vi "Example Test 3.vi"() -> ()   [LabVIEW 2014]
uses:
  <vilib>/measure/NI_MABase.lvlib
panel:
  out "error out 2":errorcluster
  out "myString":string
  out "signal out 2":waveform(dbl)
  in  "b 2":dbl=4.0
  in  "a 2":dbl=3.0
  out "signal out":waveform(dbl)
  out "error out":errorcluster
  in  "error in (no error)":errorcluster
  in  "b":dbl=2.0
  in  "a":dbl=1.0
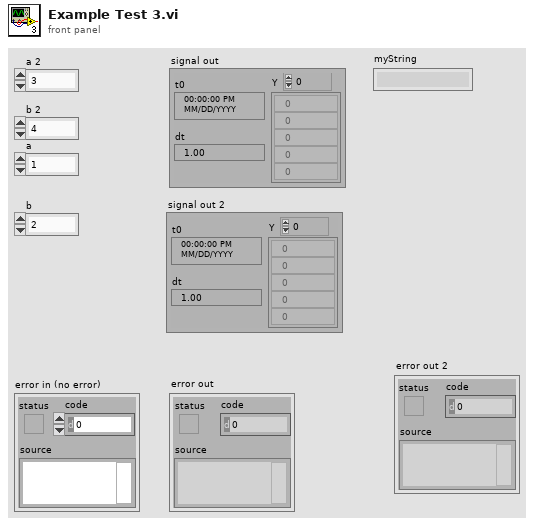
[diagram p1: front panel]
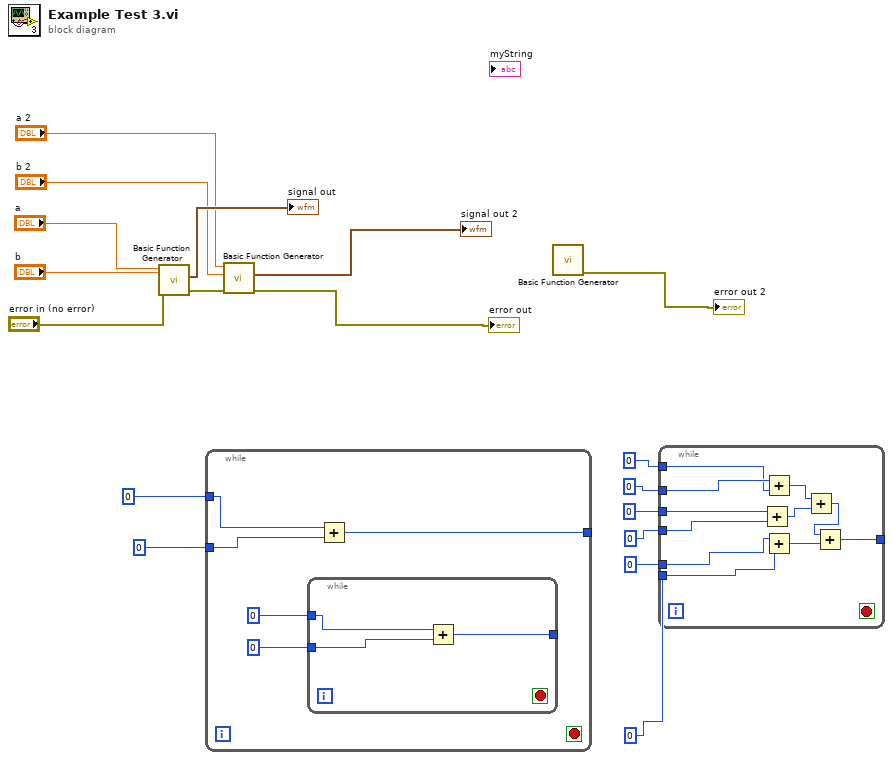
[diagram p0: block diagram]
diagram:
  n1 = call <vilib>:"Basic Function Generator.vi"("error in (no error)"="error in (no error)", "amplitude"="b", "frequency"="a") -> ("error out"=w14:errorcluster, "signal out"=→"signal out":waveform(dbl))  [unwired: 6 in, 1 out]
  n2 = while {
    tunnel: 0 -> [w23]
    tunnel: 0 ("y") -> [w22]
    tunnel: [w21] -> _
    stop <- _ stop-if-true
    n3 = while {
      tunnel: 0 -> [w26]
      tunnel: 0 ("y") -> [w25]
      tunnel: [w24] -> _
      stop <- _ stop-if-true
      n4 = Add(x=w26, y=w25) -> (x+y=w24:i32)
    }
    n5 = Add(x=w23, y=w22) -> (x+y=w21:i32)
  }
  n6 = call <vilib>:"Basic Function Generator.vi"("error in (no error)"=w14, "amplitude"="b 2", "frequency"="a 2") -> ("error out"=→"error out":errorcluster, "signal out"=→"signal out 2":waveform(dbl))  [unwired: 6 in, 1 out]
  n7 = call <vilib>:"Basic Function Generator.vi"() -> ("error out"=→"error out 2":errorcluster)  [unwired: 9 in, 2 out]
  n8 = while {
    tunnel: 0 -> [w27]
    tunnel: 0 -> [w37]
    tunnel: 0 ("y") -> [w36]
    tunnel: 0 -> [w35]
    tunnel: 0 -> [w34]
    tunnel: 0 ("y") -> [w33]
    tunnel: [w28] -> _
    stop <- _ stop-if-true
    n9 = Add(x=w36, y=w35) -> (x+y=w32:i32)
    n10 = Add(x=w37, y=w27) -> (x+y=w31:i32)
    n11 = Add(x=w34, y=w33) -> (x+y=w30:i32)
    n12 = Add(x=w31, y=w32) -> (x+y=w29:i32)
    n13 = Add(x=w29, y=w30) -> (x+y=w28:i32)
  }
